vi "8.8.3.vi"() -> ()   [LabVIEW 2018]
panel:
  in  "a정지":bool
  out "a":dbl(graph)
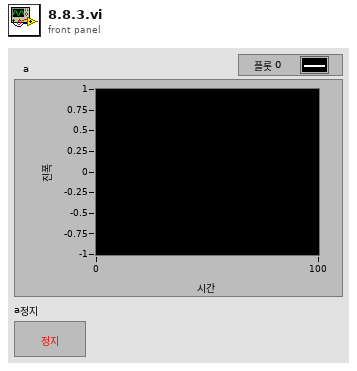
[diagram p1: front panel]
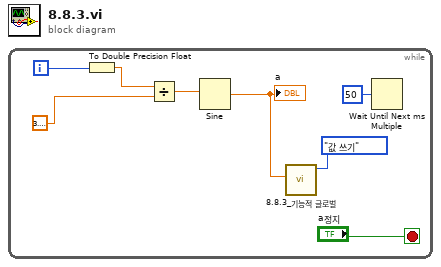
[diagram p0: block diagram]
diagram:
  n1 = while {
    i -> [w8]
    stop <- "a정지" stop-if-true
    n2 = To Double Precision Float(number=w8) -> (double precision float=w6:dbl)
    n3 = Divide(x=w6, y=3.141592653589793) -> (x/y=w4:dbl)
    n4 = Sine(x=w4) -> (sin(x)=w1:dbl)
    "a" <- w1
    n5 = call "8.8.3_기능적 글로벌.vi"("입력"=w1, "명령"=enum16{"값 쓰기", "값 읽기"}."값 쓰기") -> ()  [unwired: 1 in, 1 out]
    n6 = Wait Until Next ms Multiple(millisecond multiple=u32 50 ("ms 배수")) -> ()  [unwired: 1 out]
  }
